vi "221006_With_subVi.vi"() -> ()   [LabVIEW 2022 SP3]
uses:
  <vilib>/numeric/Random Number (Range) U64.vi
  <vilib>/numeric/sub_Random U32.vi
panel:
  out "Pt100 2":cluster{u64[], dbl[]}(graph)
  in  "B-const. 2":dbl=0.0039
  in  "A-const. 2":dbl=-5.7e-07
  in  "R0 2":dbl
  out "T in Grad 2":dbl[](array[numeric])
  out "R in Ohm 2":u64[](array[numeric])
  in  "Wertvalue 2":i32
  out "Pt100":cluster{u64[], dbl[]}(graph)
  out "T in Grad":dbl[](array[numeric])
  in  "R0":dbl
  in  "A-const.":dbl=-5.7e-07
  in  "B-const.":dbl=0.0039
  in  "Wertvalue":i32
  out "R in Ohm":u64[](array[numeric])
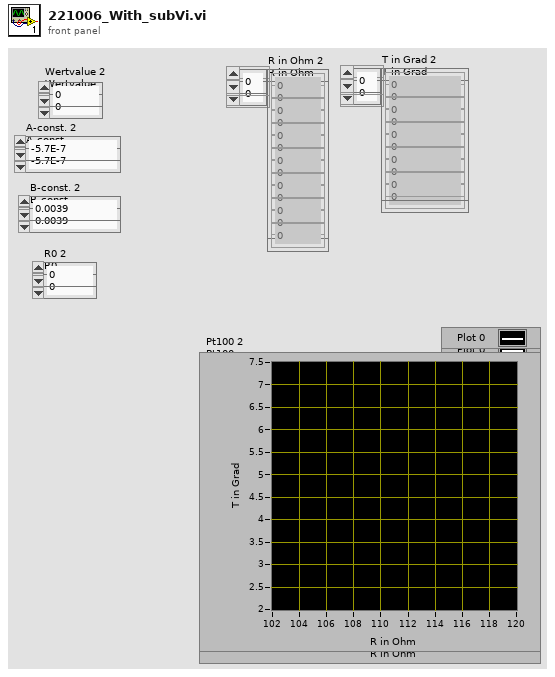
[diagram p1: front panel]
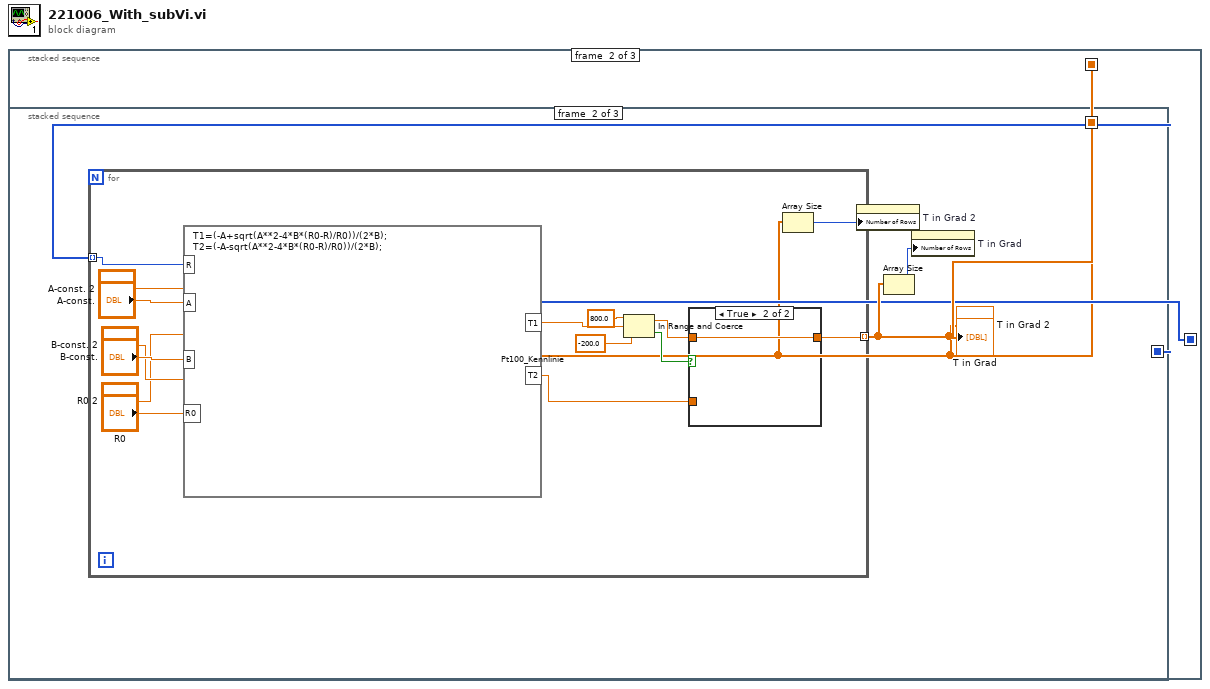
[diagram p0: block diagram]
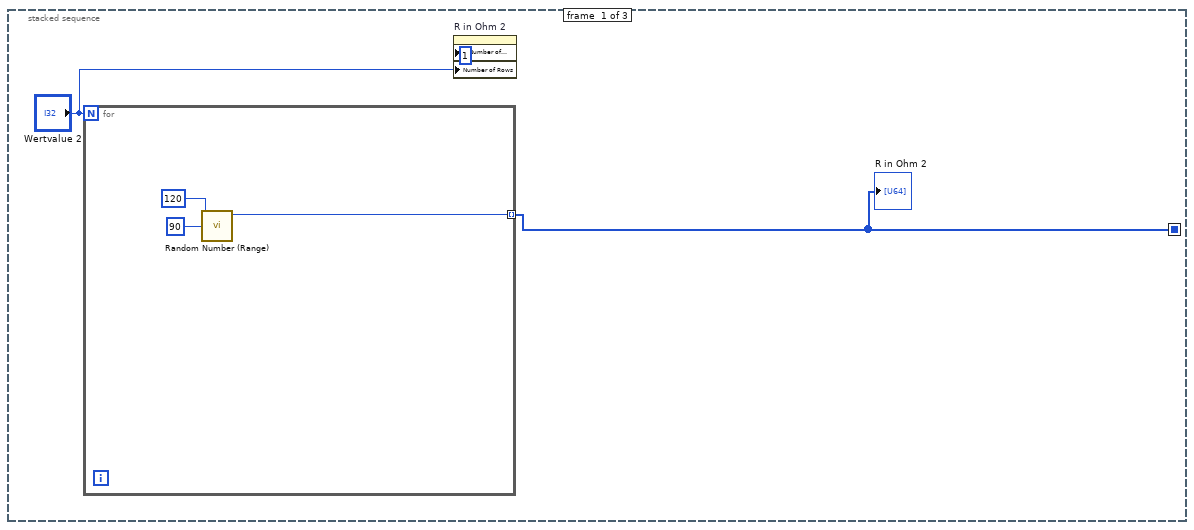
[diagram p2: hidden frame]
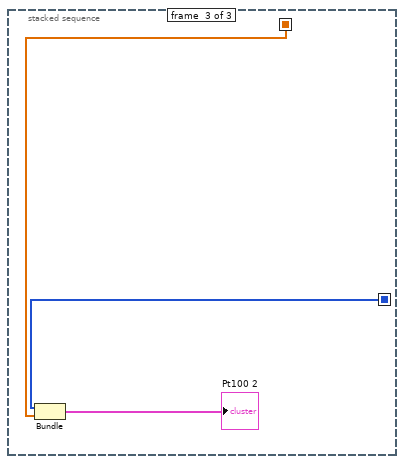
[diagram p3: hidden frame]
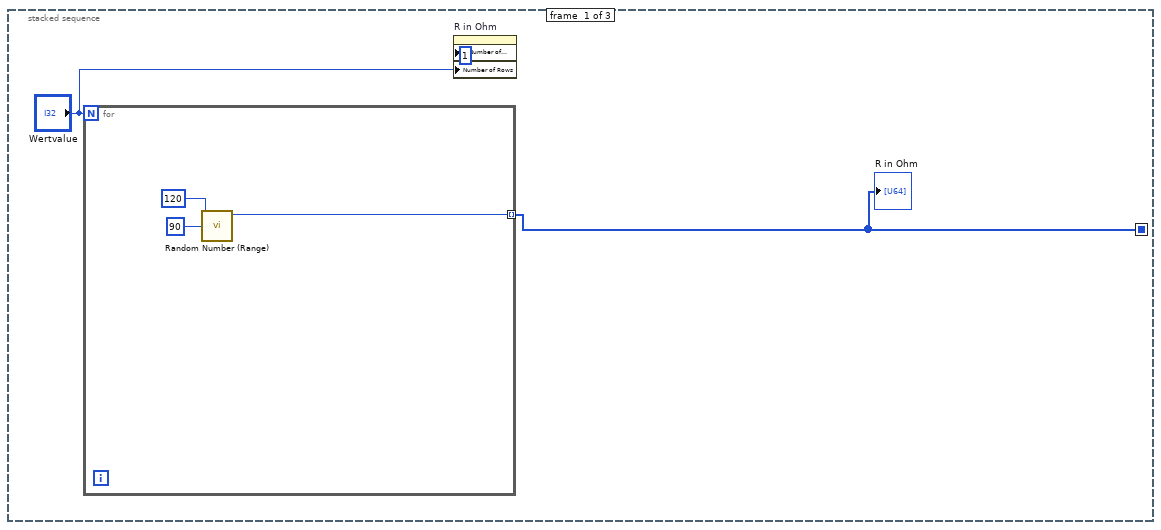
[diagram p4: hidden frame]
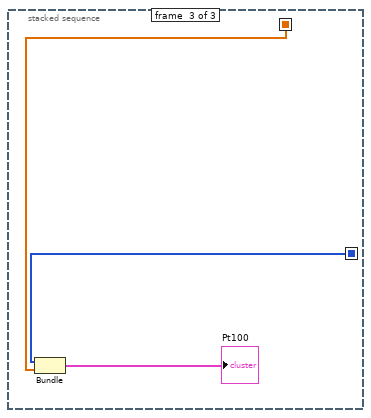
[diagram p6: hidden frame]
diagram:
  n1 = stacked-sequence {
    seq-local: [w3 _ _] -> [_ w12 w15]
    seq-local: [_ w8 _] -> [_ _ w14]
    frame #0 {
      n2 = for {
        N: "Wertvalue 2" -> [_]
        tunnel: [w4] -> w3 mode=indexing
        n3 = call-poly <vilib>:"Random Number (Range).vi"("lower bound (0)"=u64 90, "upper bound (100)"=u64 120) -> ("number"=w4:u64)  [unwired: 9 in]
      }
      "R in Ohm 2" <- w3
      n4 = property on="R in Ohm 2" class="Arr (strict)"("Number of Columns"=u32 1, "Number of Rows"="Wertvalue 2") -> ()  [unwired: 2 in, 2 out]
    }
    frame #1 {
      n5 = call "Pt100_Kennlinie.vi"("B-const. in"="B-const. 2", "R0 in"="R0 2", "A-const. in"="A-const. 2", "R in Ohm"=w12) -> ("T in Grad 2"=w8:dbl[])  [unwired: 7 in]
      "T in Grad 2" <- w8
      n6 = Array Size(array=w8) -> (size(s)=w7:i32)
      n7 = property on="T in Grad 2" class="Arr (strict)"("Number of Rows"=w7) -> ()  [unwired: 2 in, 2 out]
    }
    frame #2 {
      n8 = Bundle(w15, "T in Grad 2"=w14) -> (→"Pt100 2":cluster{u64[], "T in Grad 2":dbl[]})  [unwired: 1 in]
    }
  }
  n9 = stacked-sequence {
    seq-local: [w18 _ _] -> [_ w24 w40]
    seq-local: [_ w22 _] -> [_ _ w39]
    frame #0 {
      n10 = for {
        N: "Wertvalue" -> [_]
        tunnel: [w19] -> w18 mode=indexing
        n11 = call-poly <vilib>:"Random Number (Range).vi"("lower bound (0)"=u64 90, "upper bound (100)"=u64 120) -> ("number"=w19:u64)  [unwired: 9 in]
      }
      "R in Ohm" <- w18
      n12 = property on="R in Ohm" class="Arr (strict)"("Number of Columns"=u32 1, "Number of Rows"="Wertvalue") -> ()  [unwired: 2 in, 2 out]
    }
    frame #1 {
      n13 = for {
        tunnel: w24 -> [w35] mode=indexing
        tunnel: [w27] -> w22 mode=indexing
        n14 = formula code="T1=(-A+sqrt(A**2-4*B*(R0-R)/R0))/(2*B);\nT2=(-A-sqrt(A**2-4*B*(R0-R)/R0))/(2*B);"("R"=w35, "A"="A-const.", "B"="B-const.", "R0"="R0") -> ("T1"=w26:dbl, "T2"=w25:dbl)
        n15 = In Range and Coerce(upper limit=800.0, x=w26, lower limit=-200.0) -> (coerced(x)=w28:dbl, In Range?=w29:bool)
        n16 = case shown="True" w29 {
          tunnel: w28 -> [_ w37]
          tunnel: [w36 w37] -> w27
          tunnel: w25 -> [w36 _]
          frame False {
          }
          frame True {
          }
        }
      }
      "T in Grad" <- w22
      n17 = Array Size(array=w22) -> (size(s)=w23:i32)
      n18 = property on="T in Grad" class="Arr (strict)"("Number of Rows"=w23) -> ()  [unwired: 2 in, 2 out]
    }
    frame #2 {
      n19 = Bundle(w40, w39) -> (→"Pt100":cluster{u64[], dbl[]})  [unwired: 1 in]
    }
  }
